vi "CalculateKFOutput.vi"(8 "error in (no error)":errorcluster, 9 "Pk":dbl[][](array[numeric]), 10 "xk":dbl[](array[numeric]), 11 "MatrixCalculateOutput":T1) -> (0 "error out":errorcluster, 1 "Kalman gain":dbl[][](array[numeric]), 2 "Pk":dbl[][](array[numeric]), 3 "xk":dbl[](array[numeric]))   [LabVIEW 2014, in "AppPlugins.lvlib" / "ModelValidationPlugin.lvclass"]
uses:
  ModelValidationPlugin.lvclass
  MatrixOutput.ctl
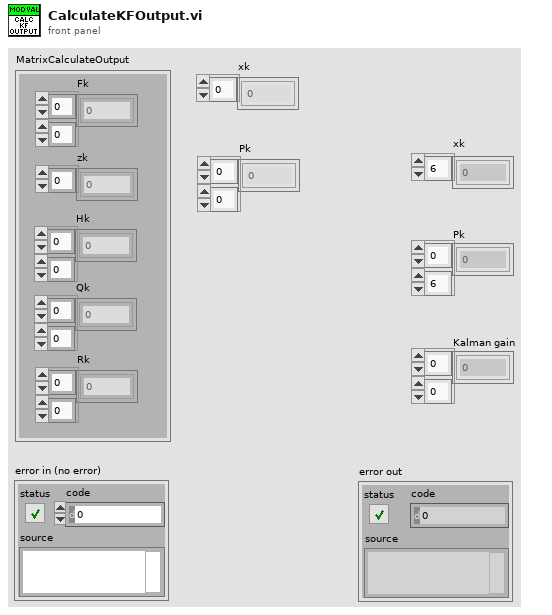
[diagram p1: front panel]
types:
  T1 = typedef "AppPlugins.lvlib/ModelValidationPlugin.lvclass/MatrixOutput.ctl" = cluster{"Fk":dbl[][], "zk":dbl[], "Hk":dbl[][], "Qk":dbl[][], "Rk":dbl[][]}
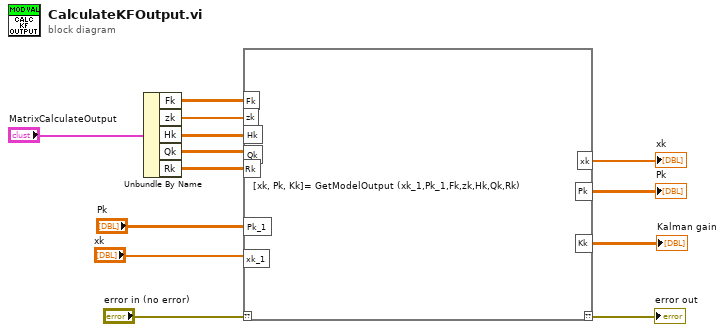
[diagram p0: block diagram]
diagram:
  n1 = Unbundle By Name("MatrixCalculateOutput") -> ("Fk"=w13:dbl[][], "zk"=w12:dbl[], "Hk"=w11:dbl[][], "Qk"=w10:dbl[][], "Rk"=w9:dbl[][])
  n2 = script code="[xk, Pk, Kk]= GetModelOutput (xk_1,Pk_1,Fk,zk,Hk,Qk,Rk)"("??"="error in (no error)", "Fk"=w13, "zk"=w12, "Hk"=w11, "Qk"=w10, "Rk"=w9, "Pk_1"="Pk", "xk_1"="xk") -> ("??"=→"error out":errorcluster, "xk"=→"xk":dbl[], "Pk"=→"Pk":dbl[][], "Kk"=→"Kalman gain":dbl[][])
